vi "OC_SBC_core.vi"(10 "value":u8 format="%02x", 11 "registers":T1={"A"=0, "X"=0, "Y"=0, "SP"=253, "PC"=0, "P"=36} {"P" format="%08b"; "PC" format="%04x"; "SP" format="%02x"; "Y" format="%02x"; "X" format="%02x"; "A" format="%02x"}) -> (3 "registers":T1={"A"=0, "X"=0, "Y"=0, "SP"=253, "PC"=0, "P"=36} {"P" format="%08b"; "PC" format="%04x"; "SP" format="%02x"; "Y" format="%02x"; "X" format="%02x"; "A" format="%02x"})   [LabVIEW 2018]
uses:
  CPU_registers.ctl
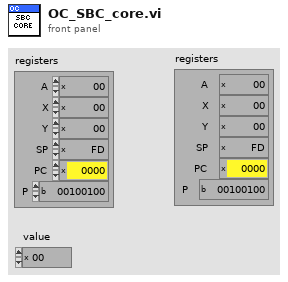
[diagram p1: front panel]
types:
  T1 = typedef "CPU_registers.ctl" = cluster{"A":u8, "X":u8, "Y":u8, "SP":u8, "PC":u16, "P":u8}
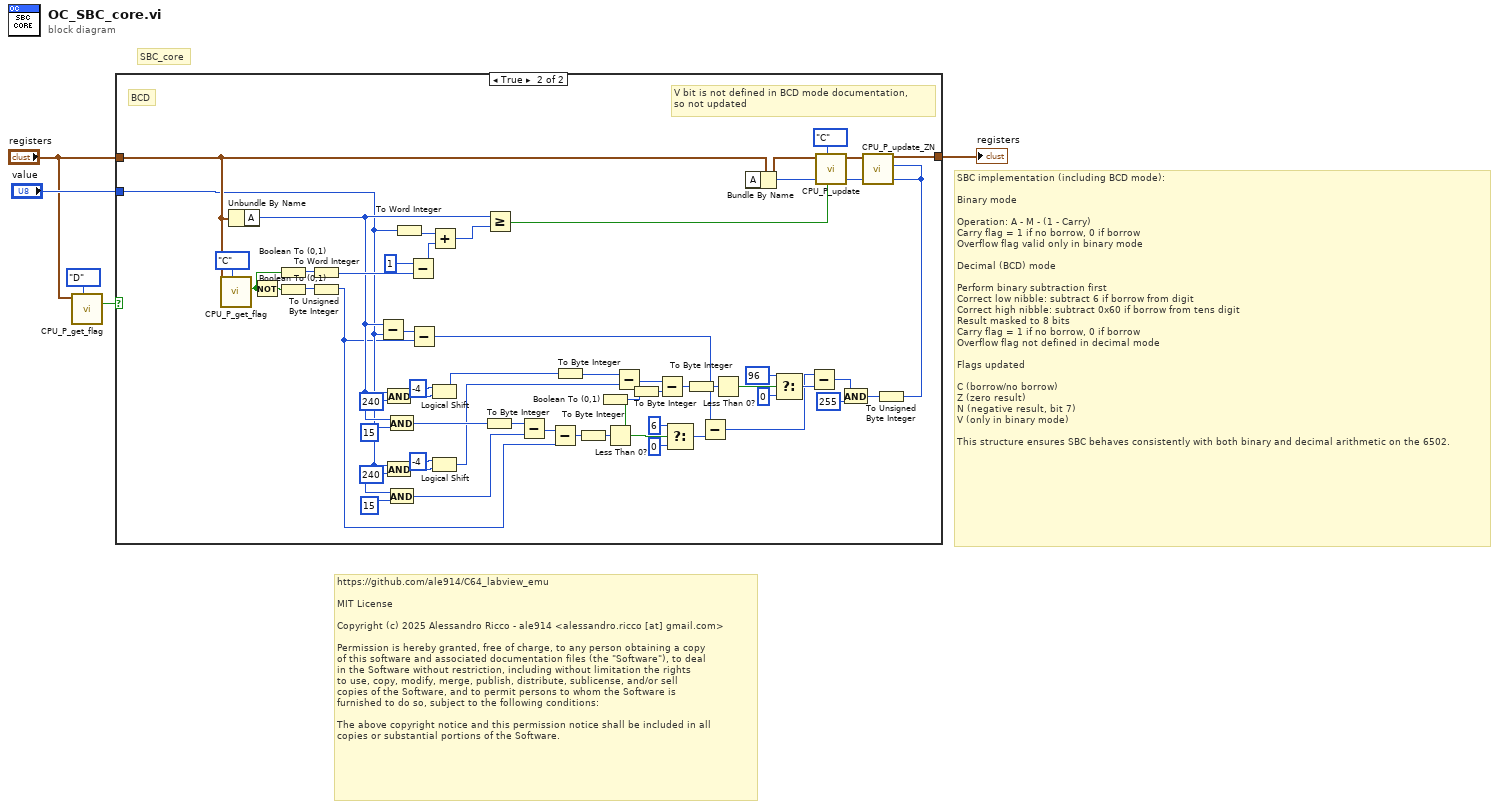
[diagram p0: block diagram]
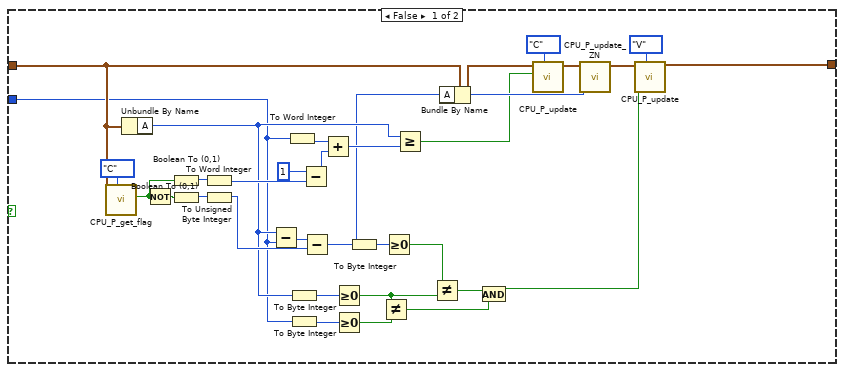
[diagram p2: hidden frame]
diagram:
  # "SBC implementation (including BCD mode):\n\nBinary mode\n\nOperation: A - M - (1 - Carry)\nCarry flag = 1 if no borrow, 0 if borrow\nOverflow flag valid only in binary mode\n\nDecimal (BCD) mode\n\nPerform binary subtraction first\nCorrect low nibble: subtract 6 if borrow from digit\nCorrect high nibble: subtract 0x60 if borrow from tens digit\nResult masked to 8 bits\nCarry flag = 1 if no borrow, 0 if borrow\nOverflow flag not defined in decimal mode\n\nFlags updated\n\nC (borrow/no borrow)\nZ (zero result)\nN (negative result, bit 7)\nV (only in binary mode)\n\nThis structure ensures SBC behaves consistently with both binary and decimal arithmetic on the 6502."
  # "https://github.com/ale914/C64_labview_emu\n\nMIT License\n\nCopyright (c) 2025 Alessandro Ricco - ale914 <alessandro.ricco [at] gmail.com>\n\nPermission is hereby granted, free of charge, to any person obtaining a copy\nof this software and associated documentation files (the \"Software\"), to deal\nin the Software without restriction, including without limitation the rights\nto use, copy, modify, merge, publish, distribute, sublicense, and/or sell\ncopies of the Software, and to permit persons to whom the Software is\nfurnished to do so, subject to the following conditions:\n\nThe above copyright notice and this permission notice shall be included in all\ncopies or substantial portions of the Software."
  # "SBC_core"
  n1 = call "CPU_P_get_flag.vi"("flag"=enum8{"C", "Z", "I", "D", "B", "V", "N"}."D", "registers"="registers") -> ("Value"=w2:bool)  [unwired: 8 in, 1 out]
  n2 = case shown="True" w2 {
    tunnel: [w30 w77] -> w5
    tunnel: "registers" -> [w29 w88]
    tunnel: "value" -> [w18 w67]
    frame False {
      n3 = call "CPU_P_get_flag.vi"("flag"=enum8{"C", "Z", "I", "D", "B", "V", "N"}."C", "registers"=w29) -> ("Value"=w6:bool)  [unwired: 8 in, 1 out]
      n4 = Unbundle By Name(w29) -> ("A"=w19:u8)
      n5 = Not(x=w6) -> (.not. x?=w25:bool)
      n6 = Boolean To (0,1)(Boolean=w6) -> (0, 1=w26:i16)
      n7 = Boolean To (0,1)(Boolean=w25) -> (0, 1=w31:i16)
      n8 = To Word Integer(number=w26) -> (16bit integer=w22:i16)
      n9 = To Unsigned Byte Integer(number=w31) -> (unsigned 8bit integer=w27:u8)
      n10 = Subtract(x=w19, y=w18) -> (x-y=w28:u8)
      n11 = To Word Integer(number=w18) -> (16bit integer=w24:i16)
      n12 = To Byte Integer(number=w19) -> (8bit integer=w17:i8)
      n13 = To Byte Integer(number=w18) -> (8bit integer=w16:i8)
      n14 = Subtract(x=i16 1, y=w22) -> (x-y=w21:i16)
      n15 = Subtract(x=w28, y=w27) -> (x-y=w9:u8)
      n16 = Add(x=w24, y=w21) -> (x+y=w20:i16)
      n17 = Greater Or Equal To 0?(x=w17) -> (x >= 0?=w14:bool)
      n18 = Greater Or Equal To 0?(x=w16) -> (x >= 0?=w15:bool)
      n19 = To Byte Integer(number=w9) -> (8bit integer=w7:i8)
      n20 = Not Equal?(x=w14, y=w15) -> (x != y?=w13:bool)
      n21 = Greater Or Equal To 0?(x=w7) -> (x >= 0?=w10:bool)
      n22 = Greater Or Equal?(x=w19, y=w20) -> (x >= y?=w8:bool)
      n23 = Not Equal?(x=w10, y=w14) -> (x != y?=w12:bool)
      n24 = Bundle By Name(cluster=w29, "A"=w9) -> (w36:T1)
      n25 = And(x=w12, y=w13) -> (x .and. y?=w11:bool)
      n26 = call "CPU_P_update.vi"("flag"=enum8{"C", "Z", "I", "D", "B", "V", "N"}."C", "Value"=w8, "registers"=w36) -> ("registers"=w35:T1)  [unwired: 8 in]
      n27 = call "CPU_P_update_ZN.vi"("value"=w9, "registers"=w35) -> ("registers"=w32:T1)  [unwired: 9 in]
      n28 = call "CPU_P_update.vi"("flag"=enum8{"C", "Z", "I", "D", "B", "V", "N"}."V", "Value"=w11, "registers"=w32) -> ("registers"=w30:T1)  [unwired: 8 in]
    }
    frame True {
      # "V bit is not defined in BCD mode documentation,\nso not updated"
      # "BCD"
      n29 = call "CPU_P_get_flag.vi"("flag"=enum8{"C", "Z", "I", "D", "B", "V", "N"}."C", "registers"=w88) -> ("Value"=w78:bool)  [unwired: 8 in, 1 out]
      n30 = Unbundle By Name(w88) -> ("A"=w72:u8)
      n31 = Not(x=w78) -> (.not. x?=w85:bool)
      n32 = Boolean To (0,1)(Boolean=w78) -> (0, 1=w86:i16)
      n33 = Boolean To (0,1)(Boolean=w85) -> (0, 1=w89:i16)
      n34 = To Word Integer(number=w86) -> (16bit integer=w82:i16)
      n35 = To Unsigned Byte Integer(number=w89) -> (unsigned 8bit integer=w62:u8)
      n36 = Subtract(x=w72, y=w67) -> (x-y=w87:u8)
      n37 = And(x=w72, y=u8 240) -> (x .and. y?=w75:u8)
      n38 = And(x=w67, y=u8 240) -> (x .and. y?=w69:u8)
      n39 = And(x=w72, y=u8 15) -> (x .and. y?=w66:u8)
      n40 = And(x=w67, y=u8 15) -> (x .and. y?=w63:u8)
      n41 = To Word Integer(number=w67) -> (16bit integer=w84:i16)
      n42 = Subtract(x=i16 1, y=w82) -> (x-y=w81:i16)
      n43 = Subtract(x=w87, y=w62) -> (x-y=w41:u8)
      n44 = Logical Shift(y=i16 -4, x=w75) -> (x << y=w55:u8)
      n45 = Logical Shift(y=i16 -4, x=w69) -> (x << y=w54:u8)
      n46 = Add(x=w84, y=w81) -> (x+y=w80:i16)
      n47 = To Byte Integer(number=w66) -> (8bit integer=w64:i8)
      n48 = Greater Or Equal?(x=w72, y=w80) -> (x >= y?=w79:bool)
      n49 = Subtract(x=w64, y=w63) -> (x-y=w65:u8)
      n50 = Subtract(x=w65, y=w62) -> (x-y=w61:u8)
      n51 = To Byte Integer(number=w55) -> (8bit integer=w56:i8)
      n52 = To Byte Integer(number=w61) -> (8bit integer=w39:i8)
      n53 = Less Than 0?(x=w39) -> (x < 0?=w53:bool)
      n54 = Boolean To (0,1)(Boolean=w53) -> (0, 1=w52:i16)
      n55 = Subtract(x=w56, y=w54) -> (x-y=w57:u8)
      n56 = To Byte Integer(number=w52) -> (8bit integer=w51:i8)
      n57 = Subtract(x=w57, y=w51) -> (x-y=w47:u8)
      n58 = Select(t=u8 6 ("y"), s=w53, f=u8 0 ("y")) -> (s? t:f=w58:u8)
      n59 = To Byte Integer(number=w47) -> (8bit integer=w38:i8)
      n60 = Subtract(x=w41, y=w58) -> (x-y=w45:u8)
      n61 = Less Than 0?(x=w38) -> (x < 0?=w46:bool)
      n62 = Select(t=u8 96 ("y"), s=w46, f=u8 0 ("y")) -> (s? t:f=w50:u8)
      n63 = Subtract(x=w45, y=w50) -> (x-y=w44:u8)
      n64 = And(x=w44, y=u8 255) -> (x .and. y?=w42:u8)
      n65 = To Unsigned Byte Integer(number=w42) -> (unsigned 8bit integer=w40:u8)
      n66 = Bundle By Name(cluster=w88, "A"=w40) -> (w92:T1)
      n67 = call "CPU_P_update.vi"("flag"=enum8{"C", "Z", "I", "D", "B", "V", "N"}."C", "Value"=w79, "registers"=w92) -> ("registers"=w91:T1)  [unwired: 8 in]
      n68 = call "CPU_P_update_ZN.vi"("value"=w40, "registers"=w91) -> ("registers"=w77:T1)  [unwired: 9 in]
    }
  }
  "registers" <- w5
